vi "Do Something.vi"(8 "error in (no error)":errorcluster, 10 "Bytes to Read":i32, 11 "Inst.Attocube-3DR in":refnum<class "Inst.Attocube-3DR.lvclass">) -> (0 "error out":errorcluster, 3 "Inst.Attocube-3DR out":refnum<class "Inst.Attocube-3DR.lvclass">)   [LabVIEW 2019, in "Inst.Attocube-3DR.lvclass"]
uses:
  Inst.Attocube-3DR.lvclass
  C:/Program Files (x86)/National Instruments/LabVIEW 2019/user.lib/LevyLab/Instrument Framework/SMOs/Instrument/Instrument.lvclass
  Typedefs/Inst.Attocube-3DR.Commands--Enum.ctl
  <userlib>/LevyLab/Instrument Framework/SMOs/Instrument/Instrument.lvclass/Instrument.ctl
  67792bfe-8e2c-4879-abc2-cb448bcec168.vi
  67792bfe-8e2c-4879-abc2-cb448bcec168.vi/e6734212-7c9e-4ce8-a442-683b18d6b7e6.vi
  <userlib>/LevyLab/Instrument Framework/SMOs/Instrument/API/Send and Receive.vi
  67792bfe-8e2c-4879-abc2-cb448bcec168.vi/d08038f8-4acd-46a3-976f-e1cbe8915b66.vi
  <userlib>/LevyLab/Instrument Framework/SMOs/Instrument/Private/Get Client Type.vi
  67792bfe-8e2c-4879-abc2-cb448bcec168.vi/e6734212-7c9e-4ce8-a442-683b18d6b7e6.vi/702ee7b8-8381-46e5-964b-170106302e58.vi
  67792bfe-8e2c-4879-abc2-cb448bcec168.vi/e6734212-7c9e-4ce8-a442-683b18d6b7e6.vi/081f70b5-aa53-4e02-9bbf-7a7e473526aa.vi
  67792bfe-8e2c-4879-abc2-cb448bcec168.vi/d08038f8-4acd-46a3-976f-e1cbe8915b66.vi/800cf9c4-7383-40cf-9bc6-eb11c7b09f2f.vi
  67792bfe-8e2c-4879-abc2-cb448bcec168.vi/d08038f8-4acd-46a3-976f-e1cbe8915b66.vi/0f5049b1-9107-4d80-b470-81422f3edf74.vi
  67792bfe-8e2c-4879-abc2-cb448bcec168.vi/d08038f8-4acd-46a3-976f-e1cbe8915b66.vi/800cf9c4-7383-40cf-9bc6-eb11c7b09f2f.vi/a0945cc9-bcdf-40fb-a272-aaee0d4097c5.vi
  67792bfe-8e2c-4879-abc2-cb448bcec168.vi/d08038f8-4acd-46a3-976f-e1cbe8915b66.vi/800cf9c4-7383-40cf-9bc6-eb11c7b09f2f.vi/98f972ea-c6c3-4374-87c9-978b47a0f9ee.vi
  <userlib>/LevyLab/Instrument Framework/SMOs/Instrument/Private/Get RC Connection Status.vi
  <userlib>/LevyLab/Instrument Framework/SMOs/Instrument/API/Enum to String.vi
  <userlib>/LevyLab/Instrument Framework/SMOs/RemoteControl/API/Send and Receive.vi
  <vilib>/Utility/Data Type/Get Type Information.vi
  <vilib>/JDP Science/JSONtext/JSON text to Variant.vi
  <userlib>/LevyLab/Instrument Framework/SMOs/Instrument/API/Instrument.GetPublicEvents.vi
  <vilib>/JDP Science/JSONtext/Variant to JSON Text.vi
  <vilib>/National Instruments/GUID Generator/Guid Generator.vi
  <userlib>/LevyLab/Instrument Framework/SMOs/Instrument/API/Instrument.MessageToProcess.vi
  <userlib>/LevyLab/Instrument Framework/SMOs/Instrument/Private/Instrument.MessageFromProcess.EventStructure.vi
  <vilib>/JDP Science/JSONtext/LVClass Serializer/JSONtext LVClass Serializer.lvclass
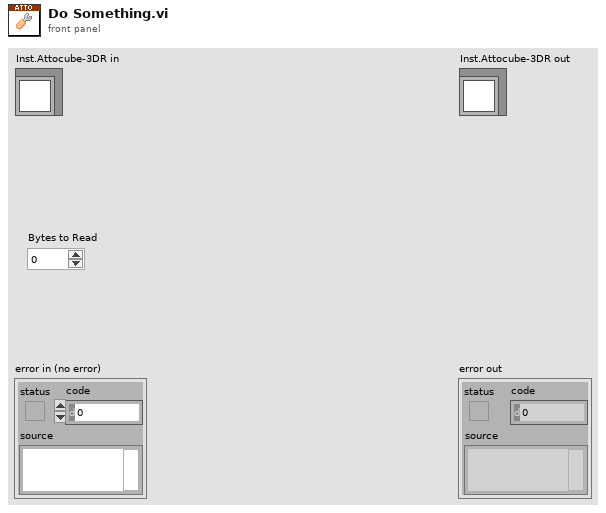
[diagram p1: front panel]
types:
  T1 = typedef "Inst.Attocube-3DR.lvclass/Inst.Attocube-3DR.Commands--Enum.ctl" = enum16{"Do Something"}
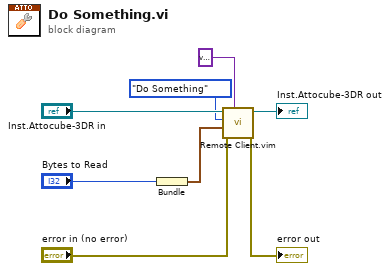
[diagram p0: block diagram]
diagram:
  n1 = Bundle("Bytes to Read"="Bytes to Read") -> (w2:cluster{"Bytes to Read":i32})  [unwired: 1 in]
  n2 = call "Remote Client.vim"("Data Out type"=variant, "error in (no error)"="error in (no error)", "params"=w2, "method"=Inst.Attocube-3DR.Commands--Enum."Do Something" ("Commands"), "Instrument in"="Inst.Attocube-3DR in") -> ("error out"=→"error out":errorcluster, "Instrument out"=→"Inst.Attocube-3DR out":refnum<class "Inst.Attocube-3DR.lvclass">)  [unwired: 3 in, 2 out]
